vi "Dropdown Selection (SubVI).vi"(1 "reference":refnum<vi>) -> (0 "element":string)   [LabVIEW 2015]
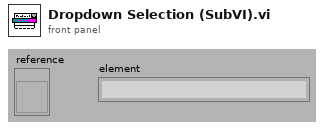
[diagram p1: front panel]
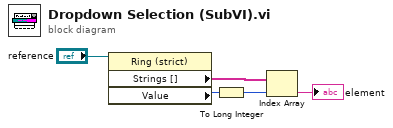
[diagram p0: block diagram]
diagram:
  n1 = property on="Property Node" class="Ring (strict)"(reference="reference") -> ("Strings []"=w5:string[], "Value"=w4:u16)  [unwired: 1 in, 2 out]
  n2 = To Long Integer(number=w4) -> (32bit integer=w3:i32)
  n3 = Index Array(array=w5, index=w3) -> (element=→"element":string)
